vi "geocoding.vi"(11 "Location":string) -> (2 "Longitude":dbl, 3 "Latitude":dbl)   [LabVIEW 2011]
uses:
  <vilib>/httpClient/LabVIEWHTTPClient.lvlib
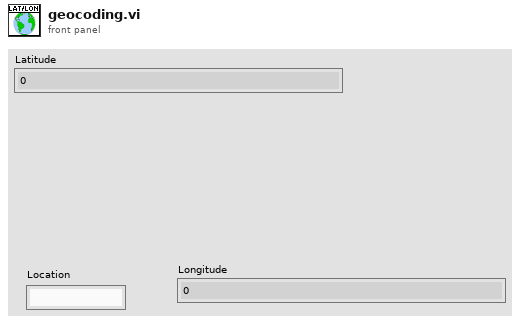
[diagram p1: front panel]
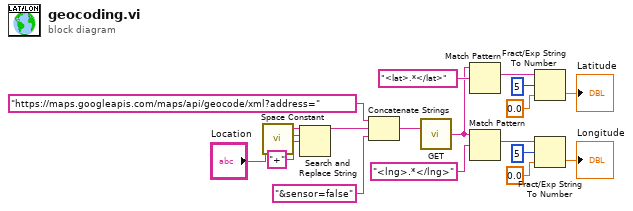
[diagram p0: block diagram]
diagram:
  n1 = call <vilib>:"Space Constant.vi"() -> ("String"=w3:string)
  n2 = Search and Replace String(input string="Location", search string=w3, replace string="+" ("replace string (\"\")")) -> (result string=w4:string)  [unwired: 5 in, 3 out]
  n3 = Concatenate Strings("https://maps.googleapis.com/maps/api/geocode/xml?address=" ("string"), w4, "&sensor=false" ("string")) -> (w1:string)
  n4 = call <vilib>:"GET.vi"("url"=w1) -> ("body"=w8:string)  [unwired: 11 in, 3 out]
  n5 = Match Pattern(string=w8, regular expression="<lat>.*</lat>") -> (match substring=w17:string)  [unwired: 1 in, 3 out]
  n6 = Match Pattern(string=w8, regular expression="<lng>.*</lng>") -> (match substring=w10:string)  [unwired: 1 in, 3 out]
  n7 = Fract/Exp String To Number(string=w17, offset=5, default (0 dbl)=0.0) -> (number=→"Latitude":dbl)  [unwired: 1 in, 1 out]
  n8 = Fract/Exp String To Number(string=w10, offset=5, default (0 dbl)=0.0) -> (number=→"Longitude":dbl)  [unwired: 1 in, 1 out]
